vi "Load Instrument.vi"(8 "error in":errorcluster, 10 "Config in":refnum<class "Config.lvclass">, 11 "Manual UI in":refnum<class "Manual UI.lvclass">) -> (0 "error out":errorcluster, 1 "Instrument":refnum<class "Instruments.lvclass">, 2 "Config out":refnum<class "Config.lvclass">, 3 "Manual UI out":refnum<class "Manual UI.lvclass">)   [LabVIEW 2019, in "Manual UI.lvlib" / "Manual UI.lvclass"]
uses:
  Project/Manual UI.lvclass
  builds/Instruments/Instruments.lvlibp/Library/Instruments.lvclass
  builds/Tools/Config.lvlibp/Config.lvclass
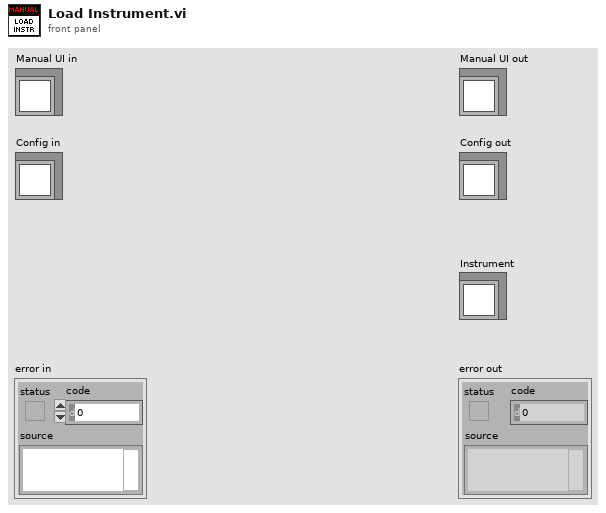
[diagram p1: front panel]
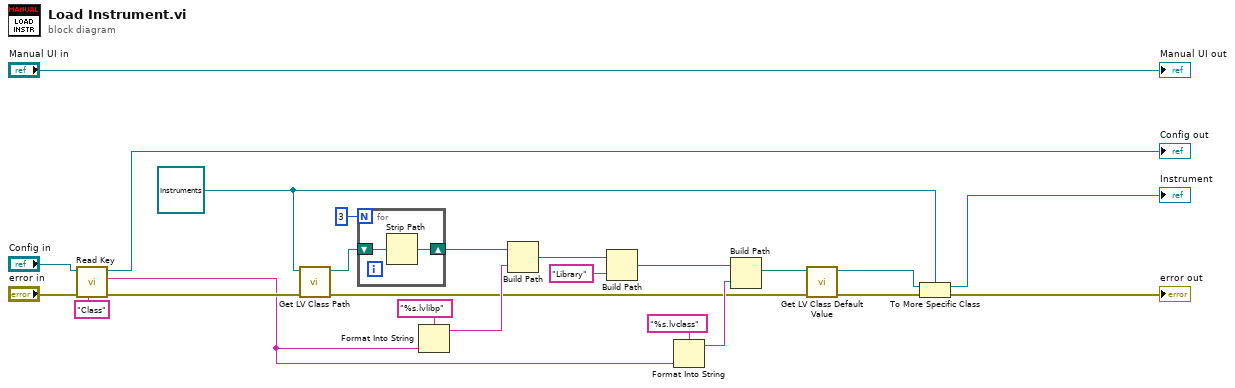
[diagram p0: block diagram]
diagram:
  w23 = refnum<class "Instruments.lvclass"> refnum ("Instruments.lvlibp:Instruments.lvclass")
  n1 = call "Read Key.vi"("Key Name"="Class", "error in"="error in", "Config in"="Config in") -> ("error out"=w4:errorcluster, "Key Value"=w3:string, "Config out"=→"Config out":refnum<class "Config.lvclass">)  [unwired: 6 in]
  n2 = call <vilib>:"Get LV Class Path.vi"("error in (no error)"=w4, "object"=w23) -> ("error out"=w9:errorcluster, "class path"=w10:path)  [unwired: 8 in]
  n3 = for {
    N: 3 -> [_]
    shift-right: [w25] -> w12
    shift-left: w10 -> [w26]
    n4 = Strip Path(path=w26) -> (stripped path=w25:path)  [unwired: 1 out]
  }
  n5 = Format Into String(format string="%s.lvlibp", w3) -> (resulting string=w14:string)  [unwired: 2 in, 1 out]
  n6 = Build Path(base path=w12, name or relative path=w14) -> (appended path=w15:path)
  n7 = Build Path(base path=w15, name or relative path="Library") -> (appended path=w17:path)
  n8 = Format Into String(format string="%s.lvclass", w3) -> (resulting string=w19:string)  [unwired: 2 in, 1 out]
  n9 = Build Path(base path=w17, name or relative path=w19) -> (appended path=w20:path)
  n10 = call <vilib>:"Get LV Class Default Value.vi"("error in (no error)"=w9, "class path"=w20) -> ("error out"=w21:errorcluster, "object"=w22:refnum<class>)  [unwired: 8 in]
  n11 = To More Specific Class(target class=w23, reference=w22, error in=w21) -> (specific class reference=→"Instrument":refnum<class "Instruments.lvclass">, error out=→"error out":errorcluster)
  "Manual UI out" <- "Manual UI in"
